vi "I2C Write Test App.vi"() -> ()   [LabVIEW 2011]
uses:
  Private/Type Defs/Interface.ctl
  Private/Device/Device.lvlib
  LVH-LINX.lvlib
panel:
  in  "Color Box":u32(colorbox)
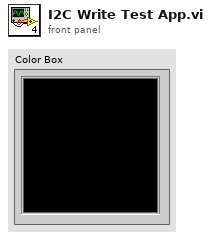
[diagram p1: front panel]
types:
  T1 = typedef "LVH-LINX.lvlib/Interface.ctl" = enum16{"Serial", "TCP"}
  T2 = typedef "LVH-LINX.lvlib/Device.lvlib/LINX Device Config.ctl" = cluster{"Interface":T1, "COM Port":refnum<visa-resource-name>, "TCP Configuration":T3, "Device Family":u8, "Device ID":u8, "Device Name":string, "TCP Ref":refnum<k5>, "Channels":T4}
  T3 = typedef "LVH-LINX.lvlib/Device.lvlib/TCP Config.ctl" = cluster{"IP Address":string, "Port":u16}
  T4 = typedef "LVH-LINX.lvlib/Channels.ctl" = cluster{"DI Channels":u8[], "DO Channels":u8[], "AI":u8[], "AO":u8[], "PWM":u8[], "QE":u8[], "UART":u8[], "I2C 2":u8[], "SPI":u8[], "CAN":u8[], "AI Ref (V)":dbl, "AO Resolution (Bits)":u8, "AO Ref (V)":dbl}
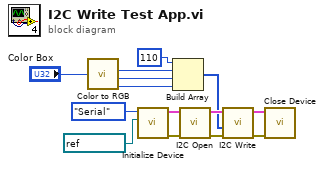
[diagram p0: block diagram]
diagram:
  n1 = call <vilib>:"Color to RGB.vi"("Color"="Color Box") -> ("R"=w5:u8, "G"=w4:u8, "B"=w3:u8)  [unwired: 1 out]
  n2 = call "Initialize Device.vi"("COM Port"=refnum<visa-resource-name> "COM5", "Interface"=Interface."Serial") -> ("Error Out"=w11:errorcluster, "LINX Device Config"=w12:T2)  [unwired: 8 in]
  n3 = Build Array(u8 110 ("element"), w5, w4, w3) -> (w2:u8[])
  n4 = call "I2C Open.vi"("Error In"=w11, "LINX Device Config"=w12) -> ("Error Out"=w9:errorcluster, "LINX Device Config"=w10:T2)  [unwired: 8 in]
  n5 = call "I2C Write.vi"("Error In"=w9, "Data"=w2, "LINX Device Config"=w10) -> ("Error Out"=w7:errorcluster, "LINX Device Config"=w8:T2)  [unwired: 7 in]
  n6 = call "Close Device.vi"("Error In"=w7, "LINX Device Config"=w8) -> ()  [unwired: 8 in, 2 out]
